vi "HEWH Trigger Draw Based On Time.vi"(7 "Station":string, 8 "Error In":errorcluster, 10 "Draw Delay":dbl, 11 "Timer Reset":bool) -> (0 "Error Out":errorcluster, 2 "Trigger Draw":bool, 3 "Elapsed Time (sec)":dbl)   [LabVIEW 2019]
uses:
  Utility/Type Definitions/UTILITY Notifier.ctl
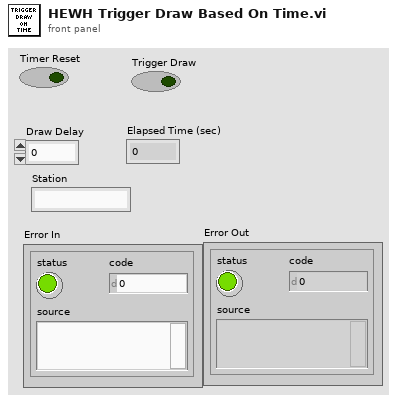
[diagram p1: front panel]
types:
  T1 = typedef "UTILITY Notifier.ctl" = enum16{"Set", "Read", "Release Ref"}
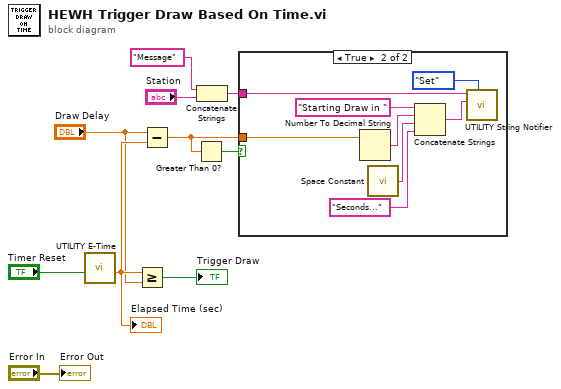
[diagram p0: block diagram]
diagram:
  n1 = call "UTILITY E-Time.vi"("Reset"="Timer Reset") -> ("Elapsed Time (sec)"=w8:dbl)  [unwired: 8 in, 2 out]
  "Elapsed Time (sec)" <- w8
  n2 = Greater Or Equal?(x=w8, y="Draw Delay") -> (x >= y?=→"Trigger Draw":bool)
  n3 = Subtract(x="Draw Delay", y=w8) -> (x-y=w9:dbl)
  n4 = Greater Than 0?(x=w9) -> (x > 0?=w10:bool)
  n5 = Concatenate Strings("Message" ("name (unnamed)"), "Station") -> (w1:string)
  n6 = case shown="True" w10 {
    tunnel: w9 -> [_ w17]
    tunnel: w1 -> [_ w11]
    frame False {
    }
    frame True {
      n7 = Number To Decimal String(number=w17) -> (decimal integer string=w15:string)  [unwired: 1 in]
      n8 = call <vilib>:"Space Constant.vi"() -> ("String"=w14:string)
      n9 = Concatenate Strings("Starting Draw in " ("Set Status"), w15, w14, "Seconds..." ("string")) -> (w12:string)
      n10 = call "UTILITY String Notifier.vi"("Status"=UTILITY_Notifier."Set", "Set Status"=w12, "name (unnamed)"=w11) -> ()  [unwired: 7 in, 2 out]
    }
  }
  "Error Out" <- "Error In"
